vi "DimIndicators.FGV_core.vi"(0 "controlRef":refnum<vi>, 1 "callBackID":i32, 2 "actions":T3, 3 "serviceName":string, 4 "queueRef":T2, 5 "error in (no error)":errorcluster, 6 "dataType":T1) -> (14 "controlRef out":refnum<vi>, 15 "callBackID out":i32, 16 "dataType out":T1, 19 "error out":errorcluster)   [LabVIEW 2014, in "DimIndicators.lvlib"]
doc: "This is a functional global variable representing the core of the DimIndicator library."
uses:
  DimIndicators.lvlib
  DimIndicators.actionType.ctl
  LVDimInterface/LVDimInterface.queue type.ctl
  DimIndicators.dataType.ctl
  LVDimInterface/LVDimInterface.dim service type.ctl
  LVDimInterface/LVDimInterface.dic_info_service_queue.vi
  LVDimInterface/LVDimInterface.lvlib
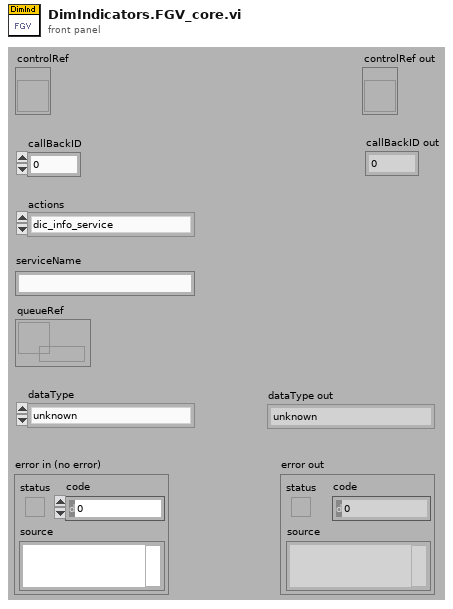
[diagram p1: front panel]
types:
  T1 = typedef "DimIndicators.lvlib/DimIndicators.dataType.ctl" = enum16{"unknown", "numeric", "numericArray", "any"}
  T2 = typedef "LVDimInterface.lvlib/LVDimInterface.queue type.ctl" = refnum<queue>
  T3 = typedef "DimIndicators.lvlib/DimIndicators.actionType.ctl" = enum16{"dic_info_service", "dic_release_service", "init", "getControlRef", "getCallbackID", "close"}
  T4 = typedef "LVDimInterface.lvlib/LVDimInterface.dim service type.ctl" = u16
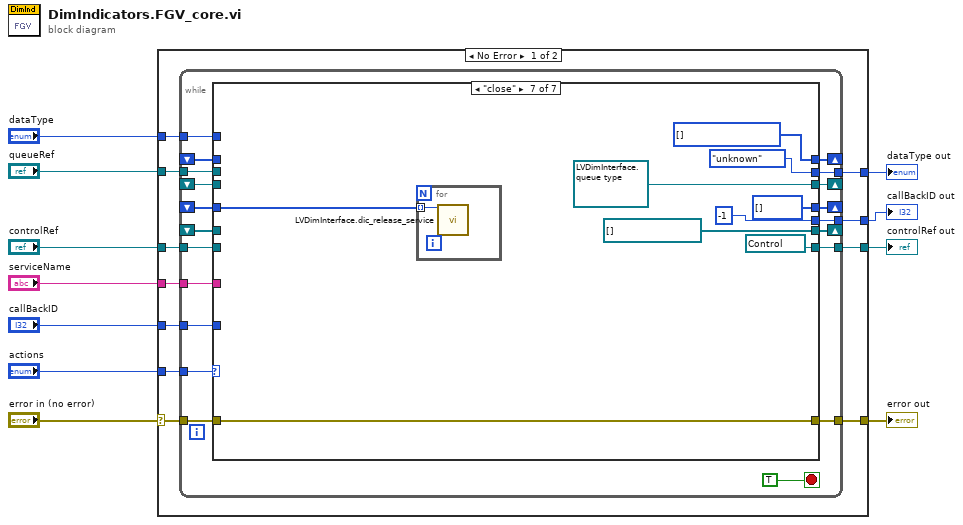
[diagram p0: block diagram]
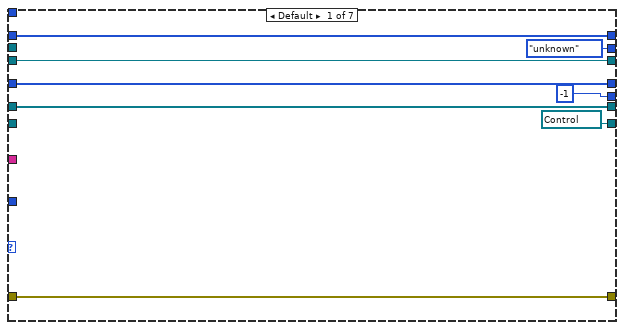
[diagram p2: hidden frame]
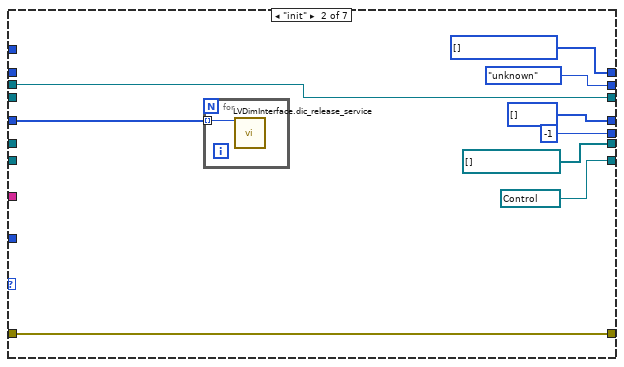
[diagram p3: hidden frame]
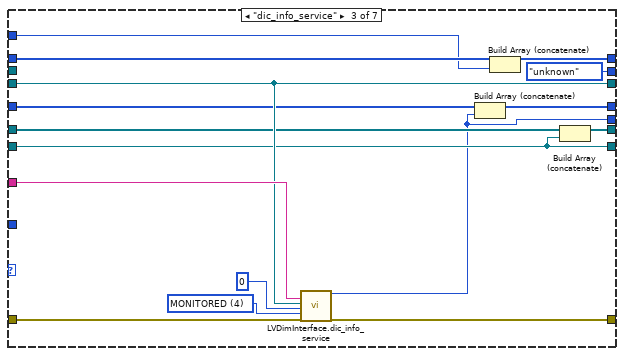
[diagram p4: hidden frame]
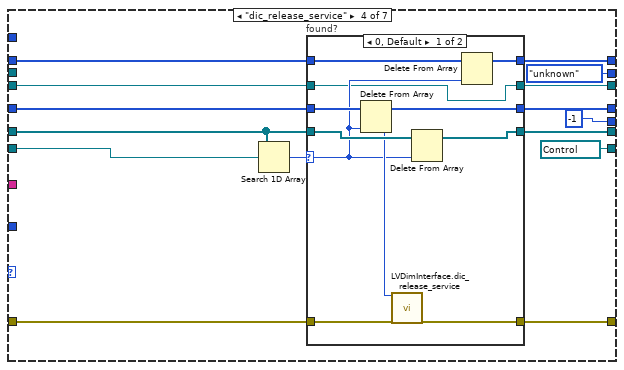
[diagram p5: hidden frame]
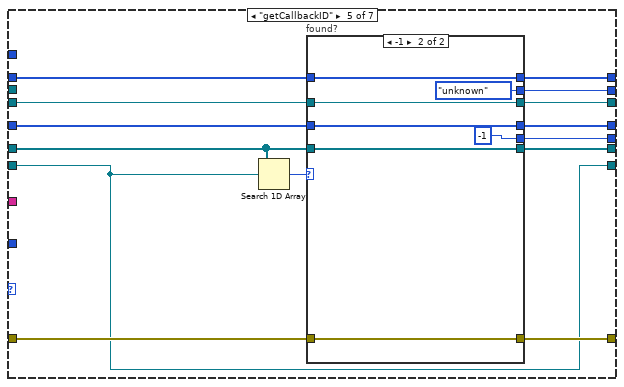
[diagram p7: hidden frame]
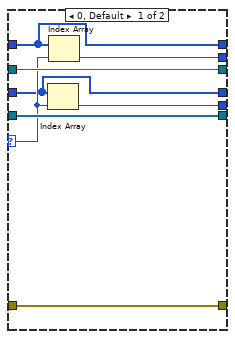
[diagram p8: hidden frame]
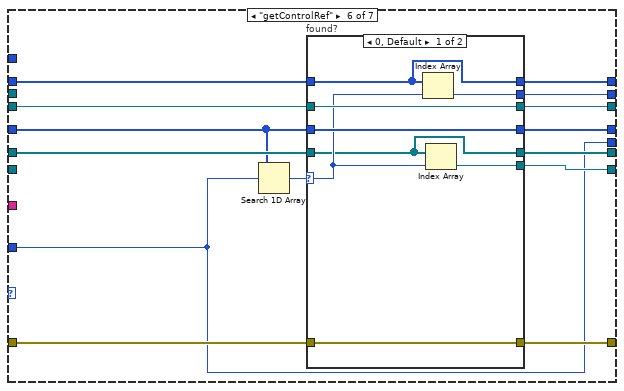
[diagram p9: hidden frame]
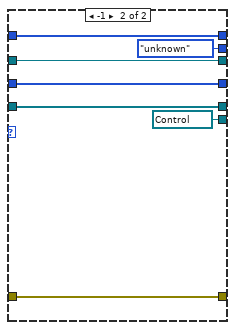
[diagram p10: hidden frame]
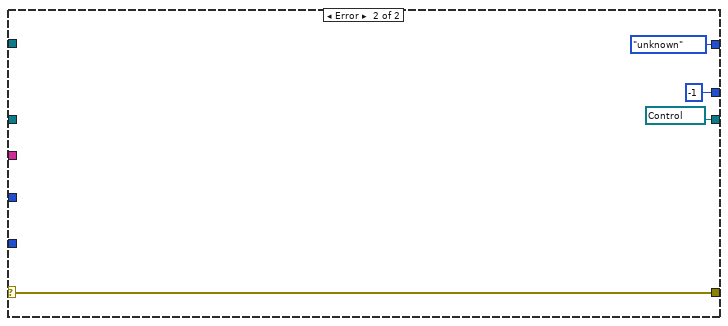
[diagram p11: hidden frame]
diagram:
  n1 = case shown="No Error" "error in (no error)" {
    selector: "error in (no error)" -> [w21 w179]
    tunnel: "actions" -> [w22 _]
    tunnel: [w20 w179] -> w10
    tunnel: "queueRef" -> [w19 _]
    tunnel: "serviceName" -> [w18 _]
    tunnel: "controlRef" -> [w17 _]
    tunnel: [w16 -1 ("callBackID")] -> w6
    tunnel: "callBackID" -> [w15 _]
    tunnel: [w14 refnum<vi> refnum ("controlRef")] -> w4
    tunnel: "dataType" -> [w13 _]
    tunnel: [w12 DimIndicators.dataType."unknown" ("dataType")] -> w2
    frame No Error {
      n2 = while {
        tunnel: w22 -> [w41]
        shift-right: [w39] -> _
        shift-left: _ -> [w40]
        tunnel: w21 -> [w38]
        tunnel: [w37] -> w20
        tunnel: w19 -> [w36]
        tunnel: w18 -> [w35]
        shift-right: [w33] -> _
        shift-left: _ -> [w34]
        shift-right: [w31] -> _
        shift-left: _ -> [w32]
        tunnel: w17 -> [w30]
        tunnel: [w29] -> w16
        tunnel: w15 -> [w28]
        tunnel: [w27] -> w14
        shift-right: [w25] -> _
        shift-left: _ -> [w26]
        tunnel: w13 -> [w24]
        tunnel: [w23] -> w12
        stop <- TRUE stop-if-true
        n3 = case shown="\"close\"" w41 {
          tunnel: [w50 w58 w73 w88 w119 w148 T2 refnum ("queueRef")] -> w39
          tunnel: w40 -> [w50 _ w73 w89 w120 w149 _]
          tunnel: w38 -> [w49 w59 w75 w84 w115 w146 w166]
          tunnel: [w49 w59 w76 w83 w114 w145 w166] -> w37
          tunnel: w36 -> [_ w58 _ _ _ _ _]
          tunnel: w35 -> [_ _ w74 _ _ _ _]
          tunnel: w34 -> [w48 w57 w70 w87 w118 w142 w174]
          tunnel: [w48 i32[] [] w69 w82 w113 w144 i32[] []] -> w33
          tunnel: w32 -> [w47 _ w68 w86 w117 w143 _]
          tunnel: [w47 refnum<vi>[] [] w67 w85 w116 w147 refnum<vi>[] []] -> w31
          tunnel: w30 -> [_ _ w62 w91 w108 _ _]
          tunnel: [-1 ("callBackID") -1 ("callBackID") w61 -1 ("callBackID") w112 w137 -1 ("callBackID")] -> w29
          tunnel: w28 -> [_ _ _ _ _ w137 _]
          tunnel: [refnum<vi> refnum ("controlRef") refnum<vi> refnum ("controlRef") w62 refnum<vi> refnum ("controlRef") w108 w141 refnum<vi> refnum ("controlRef")] -> w27
          tunnel: w26 -> [w45 _ w66 w80 w111 w140 _]
          tunnel: [w45 w53 w65 w79 w110 w139 w173] -> w25
          tunnel: w24 -> [_ _ w64 _ _ _ _]
          tunnel: [DimIndicators.dataType."unknown" ("dataType") DimIndicators.dataType."unknown" ("dataType") DimIndicators.dataType."unknown" ("dataType") DimIndicators.dataType."unknown" ("dataType") w109 w138 DimIndicators.dataType."unknown" ("dataType")] -> w23
          frame Default {
          }
          frame "init" {
            w53 = T1[] [] items=["unknown", "numeric", "numericArray", "any"]
            n4 = for {
              tunnel: w57 -> [w60] mode=indexing
              n5 = call "LVDimInterface.dic_release_service.vi"("callBackID"=w60) -> ()  [unwired: 18 in, 1 out]
            }
          }
          frame "dic_info_service" {
            w71 = T4 4 items=["ONCE_ONLY"=1, "TIMED"=2, "MONITORED"=4] ("serviceType")
            n6 = call-poly "LVDimInterface.dic_info_service.vi"("serviceName"=w74, "queueRef"=w73, "timeout [s]"=0, "serviceType"=w71, "error in (no error)"=w75) -> ("callBackID"=w61:i32, "error out"=w76:errorcluster)  [unwired: 13 in]
            n7 = Build Array (concatenate)(w70, w61) -> (w69:i32[])
            n8 = Build Array (concatenate)(w66, w64) -> (w65:T1[])
            n9 = Build Array (concatenate)(w68, w62) -> (w67:refnum<vi>[])
          }
          frame "dic_release_service" {
            n10 = Search 1D Array(1D array=w86, element=w91) -> (index of element=w90:i32)  [unwired: 1 in]
            n11 = case "found?" shown="0, Default" w90 {
              selector: w90 -> [w94 _]
              tunnel: w89 -> [w93 w106]
              tunnel: [w93 w106] -> w88
              tunnel: w87 -> [w102 w104]
              tunnel: w86 -> [w101 w105]
              tunnel: [w100 w105] -> w85
              tunnel: w84 -> [w98 w107]
              tunnel: [w97 w107] -> w83
              tunnel: [w96 w104] -> w82
              tunnel: w80 -> [w95 w103]
              tunnel: [w92 w103] -> w79
              frame 0, Default {
                n12 = Delete From Array(array=w102, index=w94) -> (deleted portion=w99:i32, array with subset deleted=w96:i32[])  [unwired: 1 in]
                n13 = call "LVDimInterface.dic_release_service.vi"("callBackID"=w99, "error in (no error)"=w98) -> ("error out"=w97:errorcluster)  [unwired: 17 in]
                n14 = Delete From Array(array=w101, index=w94) -> (array with subset deleted=w100:refnum<vi>[])  [unwired: 1 in, 1 out]
                n15 = Delete From Array(array=w95, index=w94) -> (array with subset deleted=w92:T1[])  [unwired: 1 in, 1 out]
              }
              frame -1 {
              }
            }
          }
          frame "getCallbackID" {
            n16 = Search 1D Array(1D array=w117, element=w108) -> (index of element=w121:i32)  [unwired: 1 in]
            n17 = case "found?" shown="-1" w121 {
              selector: w121 -> [w125 _]
              tunnel: w120 -> [w129 w135]
              tunnel: [w129 w135] -> w119
              tunnel: w118 -> [w122 w133]
              tunnel: w117 -> [w128 w134]
              tunnel: [w128 w134] -> w116
              tunnel: w115 -> [w127 w136]
              tunnel: [w127 w136] -> w114
              tunnel: [w122 w133] -> w113
              tunnel: [w126 -1 ("callBackID")] -> w112
              tunnel: w111 -> [w123 w131]
              tunnel: [w123 w131] -> w110
              tunnel: [w124 DimIndicators.dataType."unknown" ("dataType")] -> w109
              frame 0, Default {
                n18 = Index Array(array=w122, index=w125) -> (element=w126:i32)
                n19 = Index Array(array=w123, index=w125) -> (element=w124:T1)
              }
              frame -1 {
              }
            }
          }
          frame "getControlRef" {
            n20 = Search 1D Array(1D array=w142, element=w137) -> (index of element=w150:i32)  [unwired: 1 in]
            n21 = case "found?" shown="0, Default" w150 {
              selector: w150 -> [w153 _]
              tunnel: w149 -> [w158 w164]
              tunnel: [w158 w164] -> w148
              tunnel: w142 -> [w156 w162]
              tunnel: w143 -> [w151 w163]
              tunnel: [w151 w163] -> w147
              tunnel: w146 -> [w157 w165]
              tunnel: [w157 w165] -> w145
              tunnel: [w156 w162] -> w144
              tunnel: [w155 refnum<vi> refnum ("controlRef")] -> w141
              tunnel: w140 -> [w152 w161]
              tunnel: [w152 w161] -> w139
              tunnel: [w154 DimIndicators.dataType."unknown" ("dataType")] -> w138
              frame 0, Default {
                n22 = Index Array(array=w152, index=w153) -> (element=w154:T1)
                n23 = Index Array(array=w151, index=w153) -> (element=w155:refnum<vi>)
              }
              frame -1 {
              }
            }
          }
          frame "close" {
            w173 = T1[] [] items=["unknown", "numeric", "numericArray", "any"]
            n24 = for {
              tunnel: w174 -> [w175] mode=indexing
              n25 = call "LVDimInterface.dic_release_service.vi"("callBackID"=w175) -> ()  [unwired: 18 in, 1 out]
            }
          }
        }
      }
    }
    frame Error {
    }
  }
  "error out" <- w10
  "callBackID out" <- w6
  "controlRef out" <- w4
  "dataType out" <- w2
